vi "cmdProba.vi"() -> ()   [LabVIEW 2012]
panel:
  out "standard output":string
  out "standard error":string
  out "return code":i32
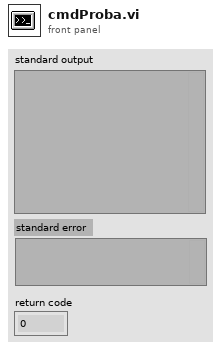
[diagram p1: front panel]
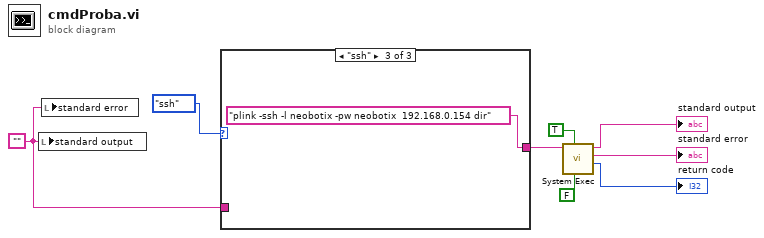
[diagram p0: block diagram]
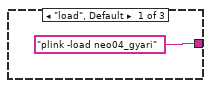
[diagram p2: hidden frame]
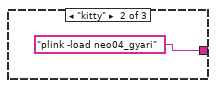
[diagram p3: hidden frame]
diagram:
  w1 = ""
  n1 = local write "standard output"(w1) -> ()
  n2 = local write "standard error"(w1) -> ()
  n3 = case shown="\"ssh\"" enum16{"load", "kitty", "ssh"}."ssh" {
    tunnel: ["plink -load neo04_gyari" ("command line 2") "plink -load neo04_gyari" ("command line 2") "plink -ssh -l neobotix -pw neobotix  192.168.0.154 dir" ("command line 2")] -> w7
    tunnel: w1 -> [_ _ _]
    frame "load", Default {
    }
    frame "kitty" {
    }
    frame "ssh" {
    }
  }
  n4 = call <vilib>:"System Exec.vi"("run minimized? (F)"=FALSE ("run minimized? 2"), "wait until completion? (T)"=TRUE ("wait until completion? 2"), "command line"=w7) -> ("return code"=→"return code":i32, "standard error"=→"standard error":string, "standard output"=→"standard output":string)  [unwired: 3 in, 3 out]
